vi "SDCP BTR Read Parameters.vi"(1 "error in (no error)":errorcluster) -> (2 "Read BTR parameters":T1[](array[typedef]), 3 "output bytes":u8[](array[numeric]), 4 "error out":errorcluster)   [LabVIEW 2020]
uses:
  Typedefs/SDCP BTR Parameter cluster.ctl
  Typedefs/SDCP BTR Parameter data type.ctl
  Typedefs/SDCP - Serial Port Control - Commands.ctl
  <vilib>/Instr/_visa.llb/VISA Flush IO Buffer Mask.ctl
panel:
  out "Time for transfer (us)":u32
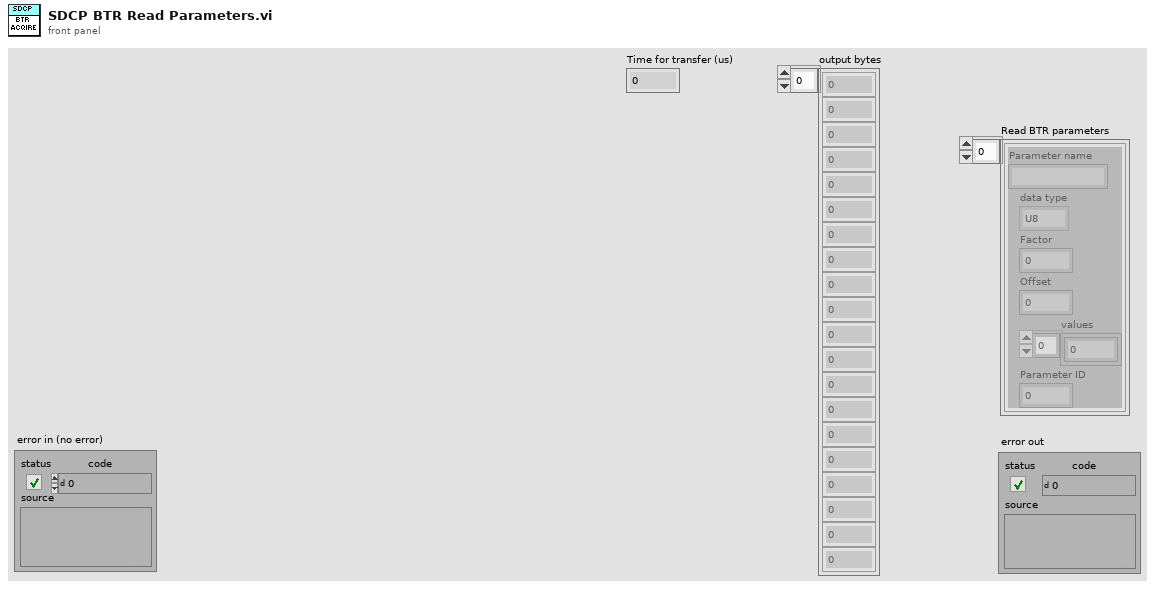
[diagram p1: front panel]
types:
  T1 = typedef "SDCP BTR Parameter cluster.ctl" = cluster{"Parameter name":string, "data type":T2, "Factor":dbl, "Offset":dbl, "values":dbl[], "Parameter ID":i32}
  T2 = typedef "SDCP BTR Parameter data type.ctl" = enum16{"U8", "I8", "U16", "I16", "U32", "I32", "F32"}
  T3 = typedef "VISA Flush IO Buffer Mask.ctl" = u16
  T4 = typedef "SDCP - Serial Port Control - Commands.ctl" = enum16{"Open", "Read", "Write", "Get instance", "Close"}
  T5 = typedef "SDCP BTR Params.ctl" = cluster{"BTR_REQ":bool, "BTR_ACK":bool, "BTR_NPAR":i32, "BTR_NTR":i32, "BTR_PIDs":u8[]}
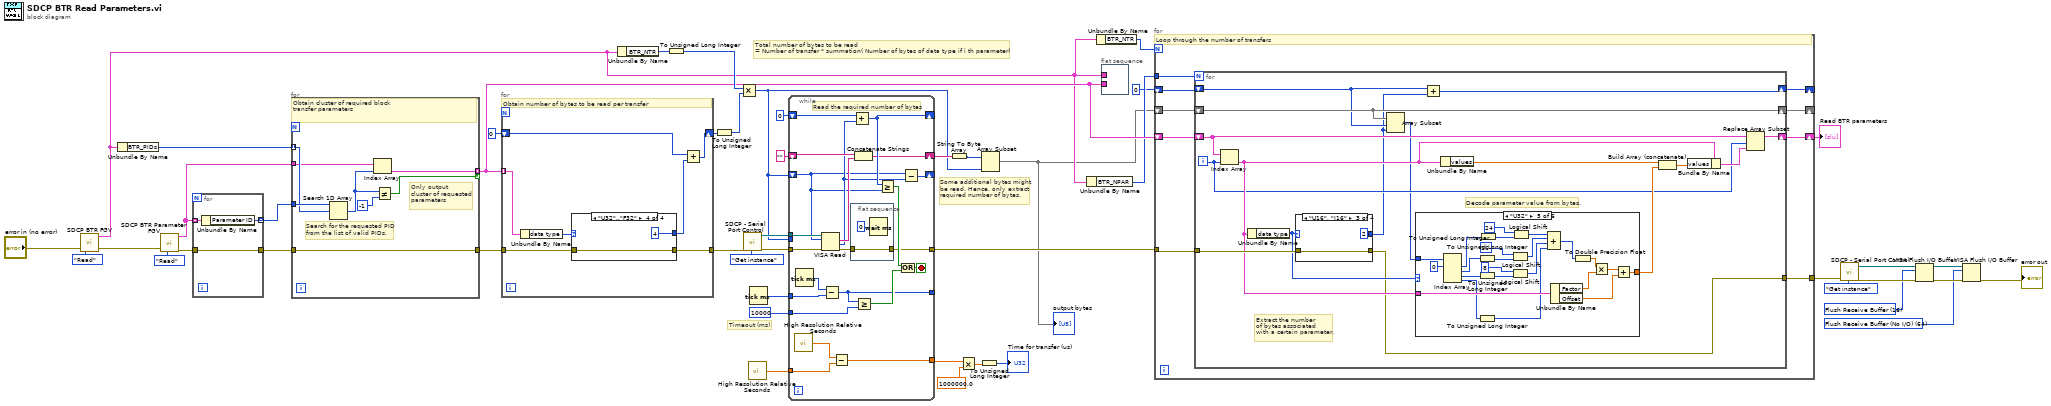
[diagram p0: block diagram]
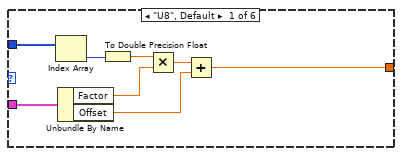
[diagram p2: hidden frame]
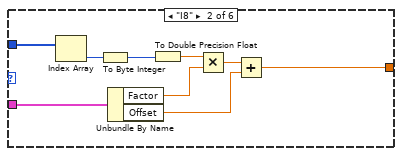
[diagram p3: hidden frame]
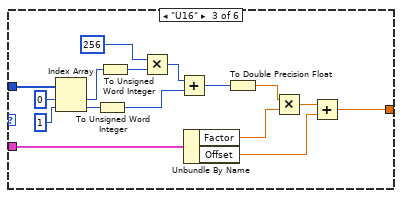
[diagram p4: hidden frame]
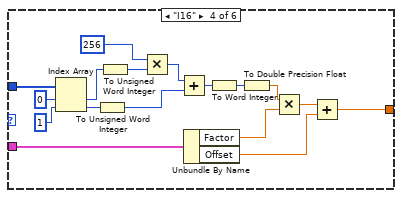
[diagram p5: hidden frame]
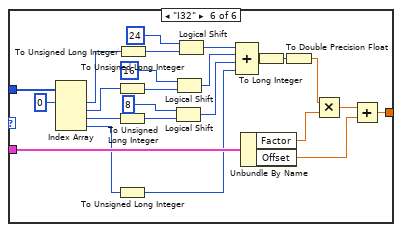
[diagram p6: hidden frame]
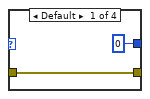
[diagram p7: hidden frame]
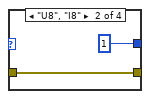
[diagram p8: hidden frame]
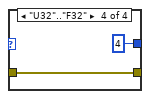
[diagram p9: hidden frame]
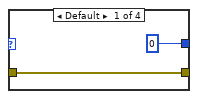
[diagram p10: hidden frame]
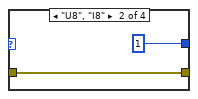
[diagram p11: hidden frame]
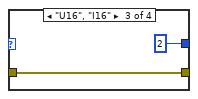
[diagram p12: hidden frame]
diagram:
  w2 = T3 64 items=["Flush Receive Buffer"=16, "Write Transmit Buffer to Device"=32, "Flush Receive Buffer (No I/O)"=64, "Flush Transmit Buffer"=128] ("Mask")
  w6 = T3 16 items=["Flush Receive Buffer"=16, "Write Transmit Buffer to Device"=32, "Flush Receive Buffer (No I/O)"=64, "Flush Transmit Buffer"=128] ("Mask")
  # "Some additional bytes might\nbe read. Hence, only extract\nrequired number of bytes."
  # "Total number of bytes to be read \n= Number of transfer * summation( Number of bytes of data type if i th parameter)"
  # "Timeout (ms)"
  n1 = call "SDCP BTR FGV.vi"("error in (no error)"="error in (no error)", "Command"=enum16{"Read", "Write"}."Read") -> ("error out"=w46:errorcluster, "out"=w20:T5)  [unwired: 2 in]
  n2 = Unbundle By Name(w20) -> ("BTR_PIDs"=w44:u8[])
  n3 = call "SDCP BTR Parameter FGV.vi"("error in (no error)"=w46, "Command"=enum16{"Load", "Read", "Write"}."Read") -> ("error out"=w43:errorcluster, "BTRP out"=w40:T1[])  [unwired: 4 in]
  n4 = for {
    tunnel: w43 -> [w51]
    tunnel: [w51] -> w42
    tunnel: w40 -> [w50] mode=indexing
    tunnel: [w49] -> w41 mode=indexing
    n5 = Unbundle By Name(w50) -> ("Parameter ID"=w49:i32)
  }
  n6 = for {
    tunnel: w44 -> [w58] mode=indexing
    tunnel: w42 -> [w52]
    tunnel: w41 -> [w59]
    tunnel: w40 -> [w57]
    tunnel: [w54] -> w21 mode=indexing if=w53
    tunnel: [w52] -> w39
    # "Only output\ncluster of requested\nparameters"
    # "Search for the requested PID\nfrom the list of valid PIDs."
    # "Obtain cluster of required block\ntransfer parameters"
    n7 = Search 1D Array(1D array=w59, element=w58) -> (index of element=w56:i32)  [unwired: 1 in]
    n8 = Index Array(array=w57, index=w56) -> (element=w54:T1)
    n9 = Not Equal?(x=w56, y=-1) -> (x != y?=w53:bool)
  }
  n10 = for {
    tunnel: w39 -> [w65]
    tunnel: w21 -> [w66] mode=indexing
    tunnel: [w63] -> w36
    shift-right: [w60] -> w27
    shift-left: 0 -> [w62]
    # "Obtain number of bytes to be read per transfer"
    n11 = Unbundle By Name(w66) -> ("data type"=w64:T2)
    n12 = case shown="\"U32\"..\"F32\"" w64 {
      tunnel: w65 -> [w68 w70 w72 w74]
      tunnel: [w68 w70 w72 w74] -> w63
      tunnel: [0 1 2 4] -> w61
      frame Default {
      }
      frame "U8", "I8" {
      }
      frame "U16", "I16" {
      }
      frame "U32".."F32" {
      }
    }
    n13 = Add(x=w62, y=w61) -> (x+y=w60:i32)
  }
  n14 = Unbundle By Name(w20) -> ("BTR_NTR"=w29:i32)
  n15 = To Unsigned Long Integer(number=w29) -> (unsigned 32bit integer=w28:u32)
  n16 = To Unsigned Long Integer(number=w27) -> (unsigned 32bit integer=w26:u32)
  n17 = Multiply(x=w28, y=w26) -> (x*y=w1:u32)
  n18 = call "SDCP - Serial Port Control.vi"("Command"=SDCP_-_Serial_Port_Control_-_Commands."Get instance", "error in (no error)"=w36) -> ("error out"=w34:errorcluster, "VISA out"=w33:refnum<visa-resource-name>)  [unwired: 6 in, 2 out]
  n19 = call <vilib>:"High Resolution Relative Seconds.vi"() -> ("relative seconds"=w15:dbl)
  n20 = Tick Count (ms)() -> (millisecond timer value=w31:u32)
  n21 = while {
    tunnel: w34 -> [w96]
    shift-right: [w93] -> _
    shift-left: 0 -> [w94]
    tunnel: w33 -> [w95]
    tunnel: w1 -> [_]
    tunnel: [w82] -> w22
    shift-right: [w91] -> w25
    shift-left: "" -> [w92]
    tunnel: w31 -> [w88]
    tunnel: 10000 -> [w87]
    tunnel: [w81] -> _
    tunnel: w15 -> [w79]
    tunnel: [w78] -> w14
    shift-right: [w76] -> _
    shift-left: w1 -> [w75]
    stop <- w86 stop-if-true
    # "Read the required number of bytes"
    n22 = call <vilib>:"High Resolution Relative Seconds.vi"() -> ("relative seconds"=w80:dbl)
    n23 = Tick Count (ms)() -> (millisecond timer value=w89:u32)
    n24 = VISA Read(VISA resource name=w95, byte count=w75, error in (no error)=w96) -> (read buffer=w90:string, return count=w77:u32, error out=w83:errorcluster)  [unwired: 1 out]
    n25 = Subtract(x=w89, y=w88) -> (x-y=w81:u32)
    n26 = Subtract(x=w80, y=w79) -> (x-y=w78:dbl)
    n27 = flat-sequence {
      tunnel: w83 -> [w98]
      tunnel: [w98] -> w82
      frame #0 {
        n28 = Wait (ms)(milliseconds to wait=u32 0) -> ()  [unwired: 1 out]
      }
    }
    n29 = Add(x=w94, y=w77) -> (x+y=w93:u32)
    n30 = Concatenate Strings(w92, w90) -> (w91:string)
    n31 = Greater Or Equal?(x=w81, y=w87) -> (x >= y?=w84:bool)
    n32 = Greater Or Equal?(x=w93, y=w75) -> (x >= y?=w85:bool)
    n33 = Or(x=w85, y=w84) -> (x .or. y?=w86:bool)
    n34 = Subtract(x=w75, y=w77) -> (x-y=w76:u32)
  }
  n35 = String To Byte Array(string=w25) -> (unsigned byte array=w24:u8[])
  n36 = Multiply(x=w14, y=1000000.0) -> (x*y=w12:dbl)
  n37 = To Unsigned Long Integer(number=w12) -> (unsigned 32bit integer=→"Time for transfer (us)":u32)
  n38 = Array Subset(array=w24, length=w1) -> (w17:u8[])  [unwired: 1 in]
  "output bytes" <- w17
  n39 = Unbundle By Name(w20) -> ("BTR_NPAR"=w19:i32)
  n40 = Unbundle By Name(w20) -> ("BTR_NTR"=w23:i32)
  n41 = flat-sequence {
    tunnel: w20 -> [_]
    tunnel: w21 -> [_]
    frame #0 {
    }
  }
  n42 = for {
    N: w23 -> [_]
    shift-right: [w104] -> _
    shift-left: w17 -> [w107]
    tunnel: w22 -> [w105]
    tunnel: w19 -> [w103]
    shift-right: [w102] -> w18
    shift-left: w21 -> [w106]
    tunnel: [w101] -> w10
    shift-right: [w99] -> _
    shift-left: 0 -> [w100]
    # "Loop through the number of transfers"
    n43 = for {
      N: w103 -> [_]
      shift-right: [w112] -> w104
      shift-left: w107 -> [w112]
      tunnel: w105 -> [w123]
      shift-right: [w116] -> w102
      shift-left: w106 -> [w117]
      tunnel: [w113] -> w101
      shift-right: [w109] -> w99
      shift-left: w100 -> [w111]
      i -> [w114]
      # "Decode parameter value from bytes."
      # "Extract the number\nof bytes associated\nwith a certain parameter."
      n44 = Index Array(array=w117, index=w114) -> (element=w119:T1)
      n45 = Unbundle By Name(w119) -> ("data type"=w122:T2)
      n46 = case shown="\"U16\", \"I16\"" w122 {
        tunnel: w123 -> [w222 w224 w226 w228]
        tunnel: [w222 w224 w226 w228] -> w113
        tunnel: [0 1 2 4] -> w110
        frame Default {
        }
        frame "U8", "I8" {
        }
        frame "U16", "I16" {
        }
        frame "U32".."F32" {
        }
      }
      n47 = Array Subset(array=w112, index=w111, length=w110) -> (w108:u8[])
      n48 = case shown="\"U32\"" w122 {
        tunnel: w119 -> [w129 w139 w155 w172 w195 w219]
        tunnel: w108 -> [w131 w140 w156 w173 w196 w220]
        tunnel: [w124 w134 w150 w167 w190 w214] -> w120
        frame "U8", Default {
          n49 = Index Array(array=w131) -> (element=w130:u8)  [unwired: 1 in]
          n50 = Unbundle By Name(w129) -> ("Factor"=w127:dbl, "Offset"=w125:dbl)
          n51 = To Double Precision Float(number=w130) -> (double precision float=w128:dbl)
          n52 = Multiply(x=w128, y=w127) -> (x*y=w126:dbl)
          n53 = Add(x=w126, y=w125) -> (x+y=w124:dbl)
        }
        frame "I8" {
          n54 = Index Array(array=w140) -> (element=w133:u8)  [unwired: 1 in]
          n55 = To Byte Integer(number=w133) -> (8bit integer=w132:i8)
          n56 = Unbundle By Name(w139) -> ("Factor"=w137:dbl, "Offset"=w135:dbl)
          n57 = To Double Precision Float(number=w132) -> (double precision float=w138:dbl)
          n58 = Multiply(x=w138, y=w137) -> (x*y=w136:dbl)
          n59 = Add(x=w136, y=w135) -> (x+y=w134:dbl)
        }
        frame "U16" {
          n60 = Index Array(array=w156, index #1=0 ("index"), index #2=1 ("index")) -> (element #1=w147:u8, element #2=w144:u8)
          n61 = To Unsigned Word Integer(number=w144) -> (unsigned 16bit integer=w142:u16)
          n62 = To Unsigned Word Integer(number=w147) -> (unsigned 16bit integer=w146:u16)
          n63 = Multiply(x=u16 256, y=w146) -> (x*y=w143:u16)
          n64 = Add(x=w143, y=w142) -> (x+y=w141:u16)
          n65 = Unbundle By Name(w155) -> ("Factor"=w153:dbl, "Offset"=w151:dbl)
          n66 = To Double Precision Float(number=w141) -> (double precision float=w154:dbl)
          n67 = Multiply(x=w154, y=w153) -> (x*y=w152:dbl)
          n68 = Add(x=w152, y=w151) -> (x+y=w150:dbl)
        }
        frame "I16" {
          n69 = Index Array(array=w173, index #1=0 ("index"), index #2=1 ("index")) -> (element #1=w164:u8, element #2=w161:u8)
          n70 = To Unsigned Word Integer(number=w161) -> (unsigned 16bit integer=w159:u16)
          n71 = To Unsigned Word Integer(number=w164) -> (unsigned 16bit integer=w163:u16)
          n72 = Multiply(x=u16 256, y=w163) -> (x*y=w160:u16)
          n73 = Add(x=w160, y=w159) -> (x+y=w158:u16)
          n74 = Unbundle By Name(w172) -> ("Factor"=w170:dbl, "Offset"=w168:dbl)
          n75 = To Word Integer(number=w158) -> (16bit integer=w157:i16)
          n76 = To Double Precision Float(number=w157) -> (double precision float=w171:dbl)
          n77 = Multiply(x=w171, y=w170) -> (x*y=w169:dbl)
          n78 = Add(x=w169, y=w168) -> (x+y=w167:dbl)
        }
        frame "U32" {
          n79 = Index Array(array=w196, index #1=0 ("index")) -> (element #1=w188:u8, element #2=w187:u8, element #3=w186:u8, element #4=w185:u8)  [unwired: 3 in]
          n80 = To Unsigned Long Integer(number=w187) -> (unsigned 32bit integer=w182:u32)
          n81 = To Unsigned Long Integer(number=w186) -> (unsigned 32bit integer=w180:u32)
          n82 = To Unsigned Long Integer(number=w185) -> (unsigned 32bit integer=w175:u32)
          n83 = To Unsigned Long Integer(number=w188) -> (unsigned 32bit integer=w184:u32)
          n84 = Logical Shift(y=i16 8, x=w180) -> (x << y=w176:u32)
          n85 = Logical Shift(y=i16 16, x=w182) -> (x << y=w177:u32)
          n86 = Logical Shift(y=i16 24, x=w184) -> (x << y=w178:u32)
          n87 = Compound Arithmetic op=ADD(w178, w177, w176, w175) -> (w174:u32)
          n88 = Unbundle By Name(w195) -> ("Factor"=w193:dbl, "Offset"=w191:dbl)
          n89 = To Double Precision Float(number=w174) -> (double precision float=w194:dbl)
          n90 = Multiply(x=w194, y=w193) -> (x*y=w192:dbl)
          n91 = Add(x=w192, y=w191) -> (x+y=w190:dbl)
        }
        frame "I32" {
          n92 = Index Array(array=w220, index #1=0 ("index")) -> (element #1=w212:u8, element #2=w211:u8, element #3=w210:u8, element #4=w209:u8)  [unwired: 3 in]
          n93 = To Unsigned Long Integer(number=w211) -> (unsigned 32bit integer=w206:u32)
          n94 = To Unsigned Long Integer(number=w210) -> (unsigned 32bit integer=w204:u32)
          n95 = To Unsigned Long Integer(number=w209) -> (unsigned 32bit integer=w199:u32)
          n96 = To Unsigned Long Integer(number=w212) -> (unsigned 32bit integer=w208:u32)
          n97 = Logical Shift(y=i16 8, x=w204) -> (x << y=w200:u32)
          n98 = Logical Shift(y=i16 16, x=w206) -> (x << y=w201:u32)
          n99 = Logical Shift(y=i16 24, x=w208) -> (x << y=w202:u32)
          n100 = Compound Arithmetic op=ADD(w202, w201, w200, w199) -> (w198:u32)
          n101 = Unbundle By Name(w219) -> ("Factor"=w217:dbl, "Offset"=w215:dbl)
          n102 = To Long Integer(number=w198) -> (32bit integer=w197:i32)
          n103 = To Double Precision Float(number=w197) -> (double precision float=w218:dbl)
          n104 = Multiply(x=w218, y=w217) -> (x*y=w216:dbl)
          n105 = Add(x=w216, y=w215) -> (x+y=w214:dbl)
        }
      }
      n106 = Add(x=w111, y=w110) -> (x+y=w109:i32)
      n107 = Unbundle By Name(w119) -> ("values"=w121:dbl[])
      n108 = Build Array (concatenate)(w121, w120) -> (w118:dbl[])
      n109 = Bundle By Name(cluster=w119, "values"=w118) -> (w115:T1)
      n110 = Replace Array Subset(array=w117, new element=w115, index=w114) -> (w116:T1[])
    }
  }
  "Read BTR parameters" <- w18
  n111 = call "SDCP - Serial Port Control.vi"("Command"=SDCP_-_Serial_Port_Control_-_Commands."Get instance", "error in (no error)"=w10) -> ("error out"=w8:errorcluster, "VISA out"=w7:refnum<visa-resource-name>)  [unwired: 6 in, 2 out]
  n112 = VISA Flush I/O Buffer(VISA resource name=w7, mask (16)=w6, error in (no error)=w8) -> (VISA resource name out=w4:refnum<visa-resource-name>, error out=w5:errorcluster)
  n113 = VISA Flush I/O Buffer(VISA resource name=w4, mask (16)=w2, error in (no error)=w5) -> (error out=→"error out":errorcluster)  [unwired: 1 out]
